vi "AssignColors.vi"(6 "Add Spaces?":bool, 8 "Front Panel":refnum<vi>, 11 "Code":refnum<vi>) -> (2 "Value":string)   [LabVIEW 2020]
uses:
  <vilib>/Utility/miscctls.llb/LVSelectionTypeDef.ctl
  ColorGlobals.vi
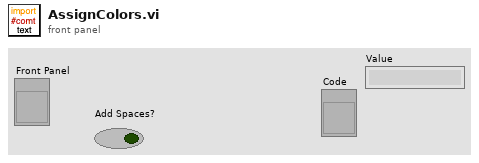
[diagram p1: front panel]
types:
  T1 = typedef "LVSelectionTypeDef.ctl" = cluster{"Selection Start":u32, "Selection End":u32}
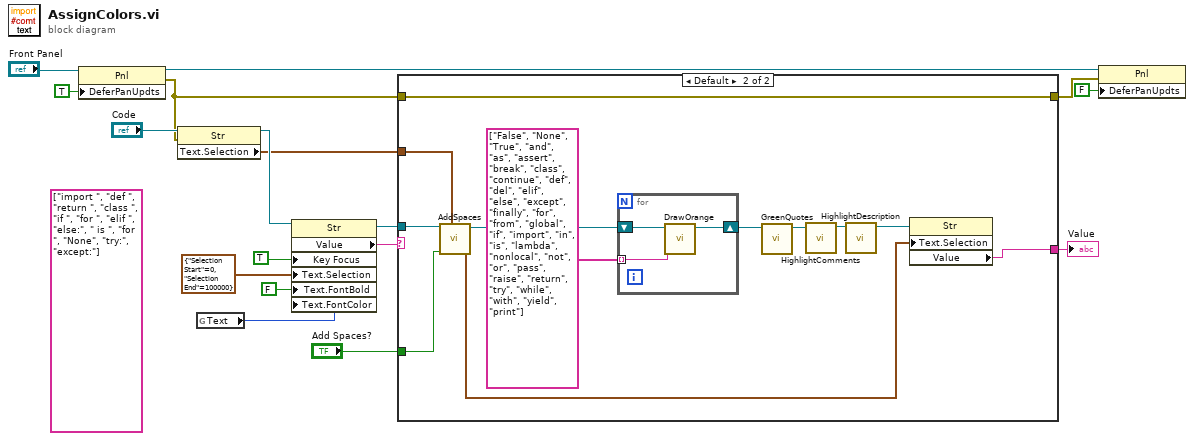
[diagram p0: block diagram]
diagram:
  (unwired) string[] ["import ", "def ", "return ", "class ", "if ", "for ", "elif ", "else:", " is ", "for ", "None", "try:", "except:"]
  n1 = property class="Pnl"(reference="Front Panel", "DeferPanUpdts"=TRUE ("Defer Panel Updates")) -> (reference out=w8:refnum<vi>, error out=w6:errorcluster)  [unwired: 1 in]
  n2 = property on="Property Node" class="Str"(reference="Code", error in=w6) -> (reference out=w14:refnum<vi>, "Text.Selection"=w13:T1)  [unwired: 1 out]
  n3 = global read "ColorGlobals.vi" "Text"() -> (w1:u32)
  n4 = property on="Property Node" class="Str"(reference=w14, "Key Focus"=TRUE, "Text.Selection"=T1 {"Selection Start"=0, "Selection End"=100000}, "Text.FontBold"=FALSE ("Text.Font:Bold"), "Text.FontColor"=w1) -> (reference out=w4:refnum<vi>, "Value"=w3:string)  [unwired: 1 in, 1 out]
  n5 = case shown="Default" w3 {
    selector: w3 -> [w19 _]
    tunnel: w4 -> [_ w25]
    tunnel: w13 -> [_ w30]
    tunnel: [w19 w29] -> w11
    tunnel: [w18 w28] -> w7
    tunnel: w6 -> [w18 w28]
    tunnel: "Add Spaces?" -> [_ w26]
    frame "" {
    }
    frame Default {
      n6 = call "AddSpaces.vi"("Text.Selection"=w30, "Add Spaces?"=w26, "String in"=w25) -> ("Cursor"=w27:cluster{u32, u32}, "String out"=w24:refnum<vi>)  [unwired: 7 in]
      n7 = for {
        shift-right: [w33] -> w20
        shift-left: w24 -> [w34]
        tunnel: string[] ["False", "None", "True", "and", "as", "assert", "break", "class", "continue", "def", "del", "elif", "else", "except", "finally", "for", "from", "global", "if", "import", "in", "is", "lambda", "nonlocal", "not", "or", "pass", "raise", "return", "try", "while", "with", "yield", "print"] -> [w32] mode=indexing
        n8 = call "DrawOrange.vi"("Expression"=w32, "String in"=w34) -> ("String out"=w33:refnum<vi>)  [unwired: 9 in]
      }
      n9 = call "GreenQuotes.vi"("String in"=w20) -> ("String out"=w21:refnum<vi>)  [unwired: 10 in]
      n10 = call "HighlightComments.vi"("String in"=w21) -> ("String out"=w22:refnum<vi>)  [unwired: 10 in]
      n11 = call "HighlightDescription.vi"("String in"=w22) -> ("String out"=w23:refnum<vi>)  [unwired: 10 in]
      n12 = property on="Property Node" class="Str"(reference=w23, "Text.Selection"=w27) -> ("Value"=w29:string)  [unwired: 1 in, 2 out]
    }
  }
  "Value" <- w11
  n13 = property class="Pnl"(reference=w8, error in=w7, "DeferPanUpdts"=FALSE ("Defer Panel Updates")) -> ()  [unwired: 2 out]
